vi "Set Voltage and Current.vi"(0 "Yokogawa WT1600 in":refnum<class "Yokogawa WT1600.lvclass">, 5 "Card #":u8, 7 "Voltage enum number":u16, 9 "Current enum number":u16, 11 "error in (no error)":errorcluster) -> (4 "Yokogawa WT1600 out":refnum<class "Yokogawa WT1600.lvclass">, 15 "error out":errorcluster)   [LabVIEW 2013, in "Universal Power Meter.lvlib" / "Yokogawa WT1600.lvlib" / "Yokogawa WT1600.lvclass"]
uses:
  Yokogawa WT1600.lvclass
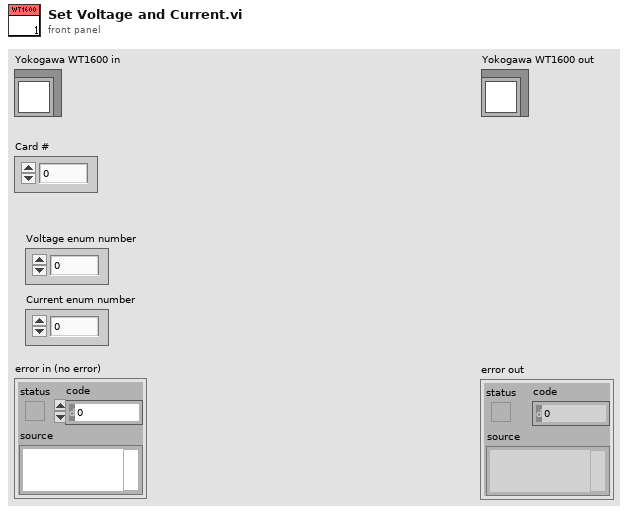
[diagram p1: front panel]
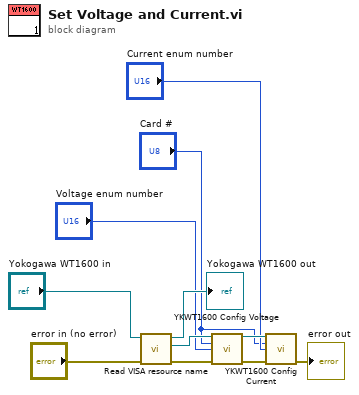
[diagram p0: block diagram]
diagram:
  n1 = call-dynamic "Read VISA resource name.vi"("error in (no error)"="error in (no error)", "Generic Instrument in"="Yokogawa WT1600 in") -> ("error out"=w6:errorcluster, "VISA resource name"=w7:refnum<visa-resource-name>, "Generic Instrument out"=→"Yokogawa WT1600 out":refnum<class "Yokogawa WT1600.lvclass">)  [unwired: 7 in]
  n2 = call <instrlib>:"YKWT1600 Config Voltage.vi"("VISA session"=w7, "Element (0: All)"="Card #", "V Range (12: 1000)"="Voltage enum number", "error in (no error)"=w6) -> ("dup VISA session"=w11:refnum<visa-resource-name>, "error out"=w10:errorcluster)  [unwired: 10 in]
  n3 = call <instrlib>:"YKWT1600 Config Current.vi"("VISA session"=w11, "Element (0: All)"="Card #", "A Range (9: 5A)"="Current enum number", "error in (no error)"=w10) -> ("error out"=→"error out":errorcluster)  [unwired: 10 in, 1 out]
